vi "TESTE_COUDE.vi"() -> ()   [LabVIEW 2012]
panel:
  out "error out":errorcluster
  out "concatenated string":string
  out "Output Message 2":string
  out "Numeric":i32
  in  "GO":bool
  in  "Angulo da rede de difração":i32=10 caption="Ângulo da Rede" min=10 max=99989 step=1
  out "parou 3":bool
  in  "stop":bool
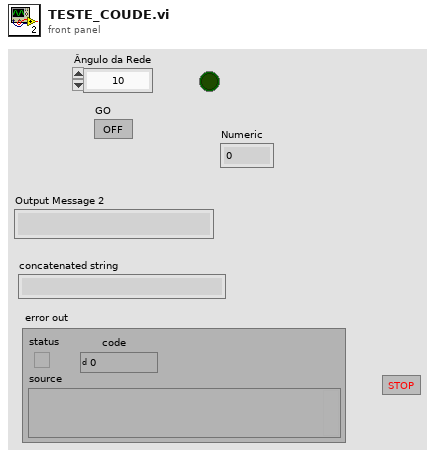
[diagram p1: front panel]
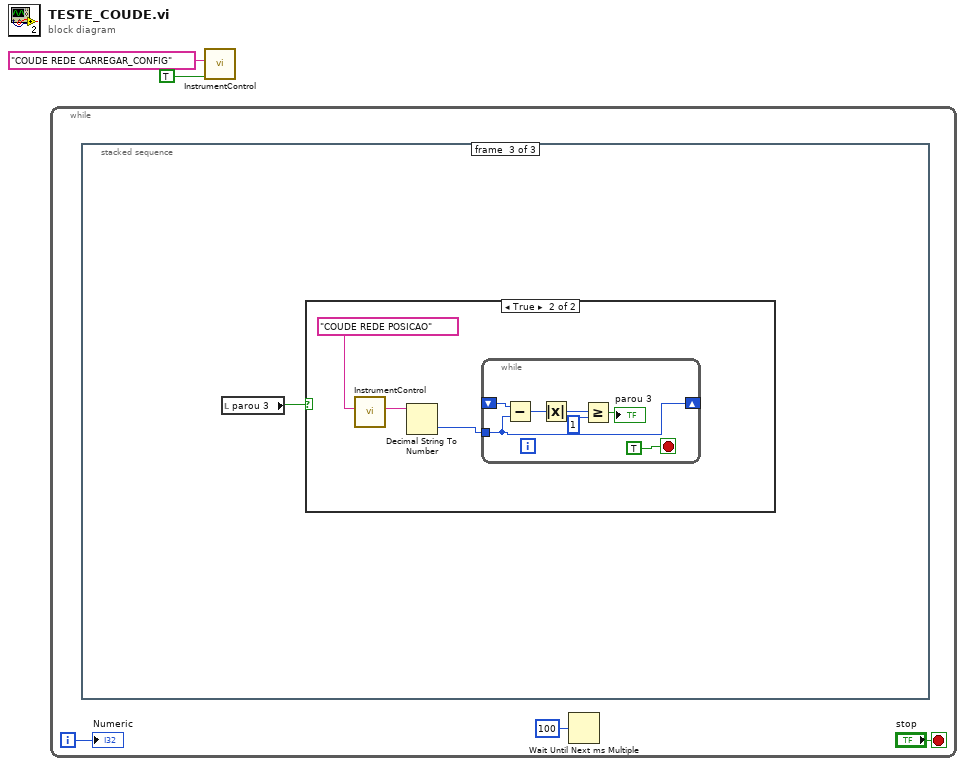
[diagram p0: block diagram]
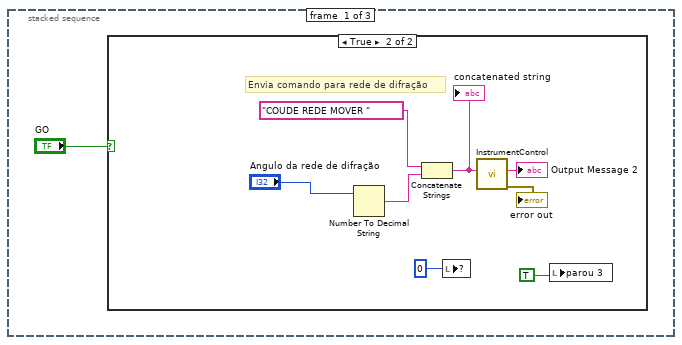
[diagram p2: hidden frame]
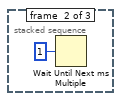
[diagram p4: hidden frame]
diagram:
  n1 = while {
    i -> [w3]
    stop <- "stop" stop-if-true
    n2 = stacked-sequence {
      frame #0 {
        n3 = case shown="True" "GO" {
          frame False {
          }
          frame True {
            # "Envia comando para rede de difração"
            n4 = Number To Decimal String(number="Angulo da rede de difração") -> (decimal integer string=w11:string)  [unwired: 1 in]
            n5 = Concatenate Strings("COUDE REDE MOVER ", w11) -> (w14:string)
            "concatenated string" <- w14
            n6 = local write item#-1(0 ("x+1")) -> ()
            n7 = call "InstrumentControl.vi"("Input Message"=w14) -> ("error out"=→"error out":errorcluster, "Output Message"=→"Output Message 2":string)  [unwired: 9 in]
            n8 = local write "parou 3"(TRUE ("parou")) -> ()
          }
        }
      }
      frame #1 {
        n9 = Wait Until Next ms Multiple(millisecond multiple=u32 1) -> ()  [unwired: 1 out]
      }
      frame #2 {
        n10 = local read "parou 3"() -> (w16:bool)
        n11 = case shown="True" w16 {
          frame False {
          }
          frame True {
            n12 = call "InstrumentControl.vi"("Input Message"="COUDE REDE POSICAO") -> ("Output Message"=w18:string)  [unwired: 9 in, 1 out]
            n13 = Decimal String To Number(string=w18) -> (number=w17:i32)  [unwired: 2 in, 1 out]
            n14 = while {
              shift-right: [w20] -> _
              shift-left: _ -> [w25]
              tunnel: w17 -> [w20]
              stop <- TRUE stop-if-true
              n15 = Subtract(x=w25, y=w20) -> (x-y=w24:i32)
              n16 = Absolute Value(x=w24) -> (abs(x)=w23:i32)
              n17 = Greater Or Equal?(x=w23, y=1) -> (x >= y?=→"parou 3":bool)
            }
          }
        }
      }
    }
    n18 = Wait Until Next ms Multiple(millisecond multiple=u32 100) -> ()  [unwired: 1 out]
    "Numeric" <- w3
  }
  n19 = call "InstrumentControl.vi"("Open VISA?"=TRUE, "Input Message"="COUDE REDE CARREGAR_CONFIG") -> ()  [unwired: 8 in, 2 out]
